vi "FPGA cRIOMain_v5.vi"() -> ()   [LabVIEW 2019]
doc: "Main FPGA VI\nUse the bitfile generated by this VI in the real-time code.\n\nv5: Use 16-pt MA filter in AI loop"
uses:
  TypeDefs/AO mode TabCtrl.ctl
  TypeDefs/SamplingModeEnum.ctl
  TypeDefs/AI_channelEnum.ctl
  <vilib>/rvi/Emulation/niFpgaGetClockAttributes.vi
  <vilib>/rvi/Emulation/niFpgaSctlEmulationGetInTimedLoop.vi
  <vilib>/rvi/Emulation/niFpgaEmulationReportErrorSimple.vi
  <vilib>/rvi/eio/common/nirviEmuTemplateMethod_errors.vi
  <vilib>/rvi/Emulation/niFpgaEmulationIsFPGAContextNoSignature.vi
  <vilib>/rvi/DataTransferAndStorage/Container/Common/niFpgaContainerGetUniqueNameForEmu.vi
  <vilib>/rvi/Memory/Memory_Emulation/niFpgaMemoryEmulationCacheClearOnFirstRun.vi
  <vilib>/rvi/Memory/Memory_Emulation/nirvimemoryEmulationManagerCache_MakeExclusive.vi
  <vilib>/rvi/Memory/Memory_Emulation/niFpgaMemoryEmulationValidateCache.vi
  <vilib>/rvi/Memory/Memory_Emulation/nirvimemoryEmulationManagerCache_InsertValue.vi
  <vilib>/Utility/error.llb/Clear Errors.vi
  <vilib>/rvi/Memory/Memory_Emulation/nirvimemoryEmulationManagerCache_ReleaseExclusive.vi
  <vilib>/rvi/Memory/Memory_Emulation/nirvimemoryEmulationManagerCache_GetValue.vi
  <vilib>/rvi/Memory/Memory_Emulation/nirvimemoryEmulationManagerCache_SetValue.vi
  <vilib>/rvi/Emulation/niFpgaProcessEmulError.vi
  <vilib>/rvi/Emulation/niFpgaCriticalErrorInLSC.vi
  <vilib>/rvi/errors/niFpgaSetErrorForExecOnDevCompSimple.vi
  <vilib>/rvi/eio/common/nirviEmuReportErrorAndStop.vi
  <vilib>/rvi/FIFO/Fifo_Resource/nirvififoEmulationSetSize.vi
  <vilib>/rvi/FIFO/Fifo_Resource/nirviFifoEmulationQueueMgr.vi
  <instcachedir>/0/nirviFifoEmulationQueueMgr_E5CAEC123FF24DC58D834DCA3CDAA9B5.lvgen/nirviFifoEmulationQueueMgr_E5CAEC123FF24DC58D834DCA3CDAA9B5_006.vi
  <vilib>/rvi/FIFO/Fifo_Resource/nirvififoEmulationCreateLock.vi
  <vilib>/rvi/FIFO/Fifo_Resource/nirvififoEmulationObtainLock.vi
  <vilib>/rvi/FIFO/Fifo_Resource/nirvififoEmulationReleaseLock.vi
  <vilib>/rvi/occurrence/nirviWaitOnOccurrenceBase.vi
  <vilib>/rvi/errors/nirviReportUnexpectedCaseInternalError.vi
  <vilib>/rvi/errors/nirviReportUnexpectedCaseInternalError (U32).vi
  <vilib>/rvi/FIFO/Fifo_Resource/nirvififoEmulationDetermineInputValidOut.vi
  <vilib>/eio/EIONode/EIONode.xnode
  <vilib>/rvi/DataTransferAndStorage/Container/XNode/niFpgaContainer.xnode
  <vilib>/rvi/DataTransferAndStorage/Register/Emulation/niFpgaRegisterEmulation.vi
  <vilib>/rvi/FIFO/Fifo_Resource/nirvififoEmulationRead.vi
  <vilib>/rvi/Analysis/measure/butterworth/XNode/niFpgaButterworthFilter.xnode
  <vilib>/rvi/FXPMathLib/FxpMul/XNode/nifxpmath_Multiplier.xnode
  <vilib>/rvi/FIFO/Fifo_Resource/nirvififoEmulationWrite.vi
  FPGA functions/FPGA functions.lvlib
  <vilib>/rvi/FXPMathLib/sim/FxpSim.dll
panel:
  out "AI Processing\nLoop Rate to high?":bool
  in  "AI Process Time [ticks]":u32=121
  in  "Select Channel":T1
  out "Unable to\nsample at desired\nSample Rate?":bool
  out "Processing Loop time [ticks]":u32
  in  "Scaled Butterworth Coeffs":i32[](array[numeric])=[-1036986264, 2110353124, 93741, -1058362983, 2131726043, 94691]
  in  "Sampling Mode":T2
  in  "AO mode":T3
  in  "AO Out [V]":fxp<+/-,18,5> format="%#.6g"
  in  "AO enable?":bool
  out "AI In [V]":fxp<+/-,26,5> format="%#.6g"
  out "FPGA AO DMA\nOverflow?":bool
  out "Int. Output":fxp<+/-,20,5> format="%.17g"
  out "Raw AI Input":fxp<+/-,24,5> format="%.21g"
  in  "Sample Time [ticks]":u32=121
  out "AO Loop time [ticks]":u32
  out "AI Loop time [ticks]":u32
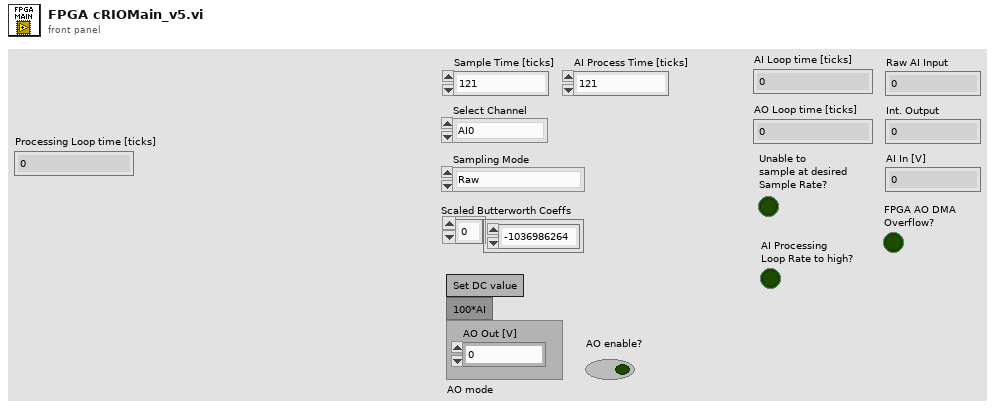
[diagram p1: front panel]
types:
  T1 = typedef "AI_channelEnum.ctl" = enum16{"AI0", "AI1", "AI2", "AI3"}
  T2 = typedef "SamplingModeEnum.ctl" = enum16{"Raw", "M64 (ReSpl)", "M128 (ReSpl)", "4pt MA (AI) + M64 (ReSpl)", "LPF (Proc.)", "4pt MA (AI) + LPF (Proc.)", "4pt MA (Proc.) + LPF (Proc.)"}
  T3 = typedef "AO mode TabCtrl.ctl" = enum32{"Set DC value", "100*AI"}
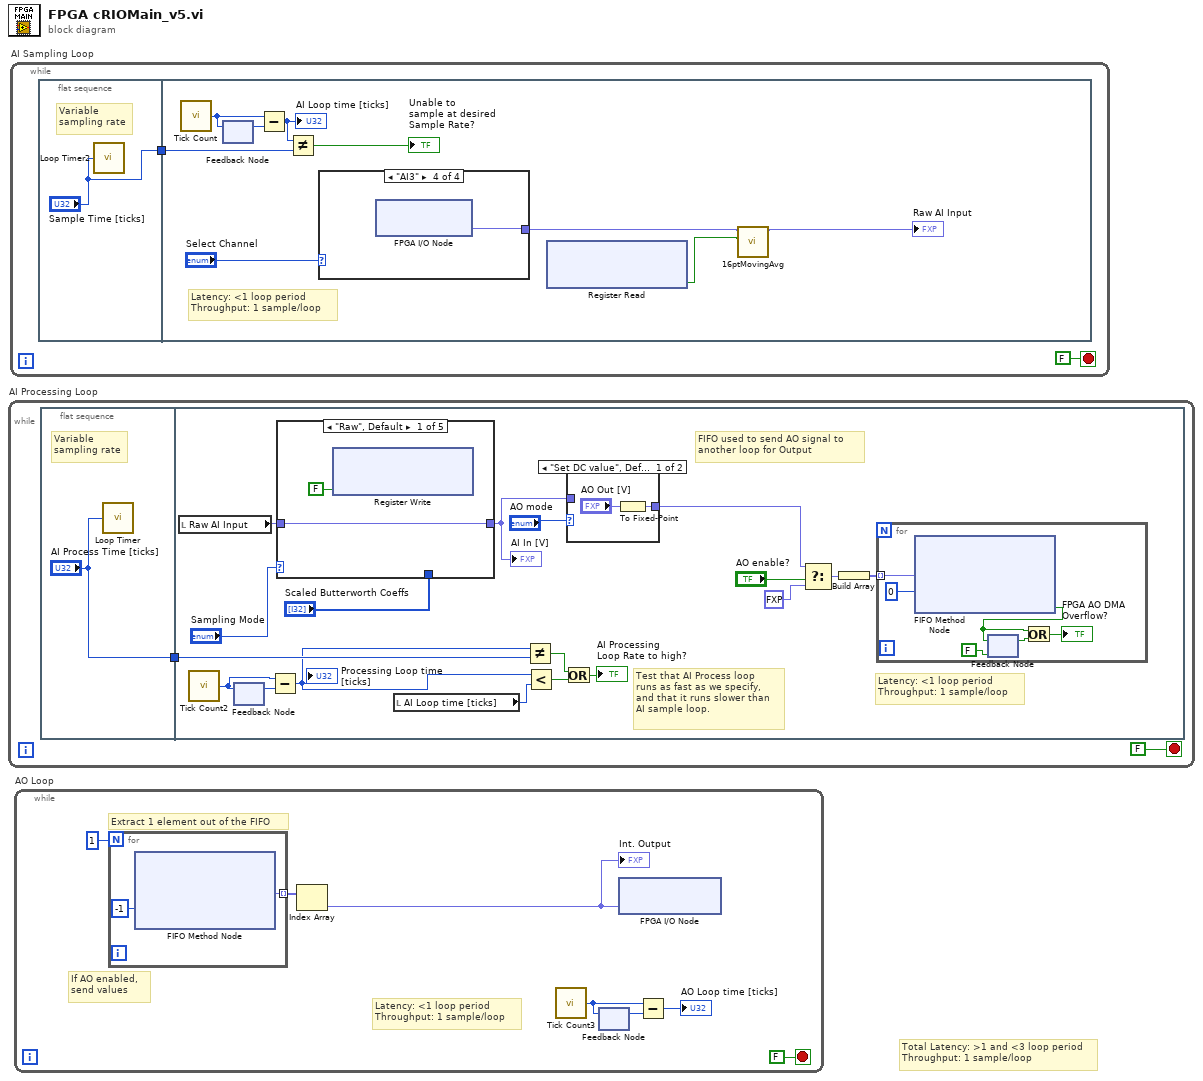
[diagram p0: block diagram]
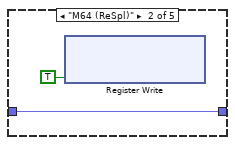
[diagram p2: hidden frame]
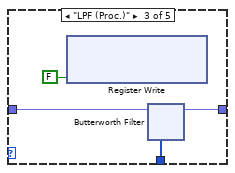
[diagram p3: hidden frame]
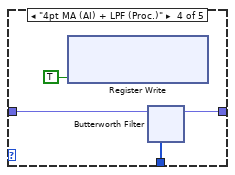
[diagram p4: hidden frame]
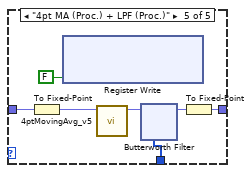
[diagram p5: hidden frame]
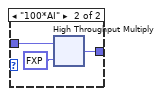
[diagram p6: hidden frame]
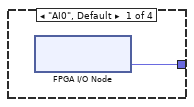
[diagram p7: hidden frame]
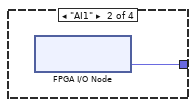
[diagram p8: hidden frame]
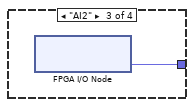
[diagram p9: hidden frame]
diagram:
  # "Total Latency: >1 and <3 loop period\nThroughput: 1 sample/loop"
  n1 = while "AI Processing Loop" {
    stop <- FALSE stop-if-true
    n2 = flat-sequence {
      tunnel: ["AI Process Time [ticks]"] -> w1
      tunnel: w1 -> [w5]
      frame #0 {
        # "Variable\nsampling rate"
        n3 = call "Loop Timer"("Count(Ticks)"="AI Process Time [ticks]") -> ()  [unwired: 1 out]
      }
      frame #1 {
        # "Test that AI Process loop\nruns as fast as we specify,\nand that it runs slower than \nAI sample loop."
        # "Latency: <1 loop period\nThroughput: 1 sample/loop"
        # "FIFO used to send AO signal to \nanother loop for Output"
        n4 = local read "Raw AI Input"() -> (w9:fxp<+/-,24,5>)
        n5 = call "Tick Count2"() -> ("Tick Count(Ticks)"=w20:u32)
        n6 = feedback #1() -> (w21:u32)  [unwired: 1 in]
        n7 = feedback-in #1(w20) -> ()
        n8 = Subtract(x=w20, y=w21) -> (x-y=w4:u32)
        "Processing Loop time [ticks]" <- w4
        n9 = case shown="\"Raw\", Default" "Sampling Mode" {
          tunnel: "Scaled Butterworth Coeffs" -> [_ _ w29 w41 w56]
          tunnel: [w22 w24 w28 w40 w50] -> w18
          tunnel: w9 -> [w22 w24 w26 w38 w53]
          frame "Raw", Default {
            n10 = xnode ("Register Write")("Data"=FALSE) -> ()  [unwired: 1 in, 1 out]
          }
          frame "M64 (ReSpl)" {
            n11 = xnode ("Register Write")("Data"=TRUE) -> ()  [unwired: 1 in, 1 out]
          }
          frame "LPF (Proc.)" {
            n12 = xnode ("Register Write")("Data"=FALSE) -> ()  [unwired: 1 in, 1 out]
            n13 = xnode "Butterworth Filter"("input data"=w26, "scaled coefficients"=w29) -> ("output data"=w28:fxp<+/-,24,5>)  [unwired: 1 in]
          }
          frame "4pt MA (AI) + LPF (Proc.)" {
            n14 = xnode ("Register Write")("Data"=TRUE) -> ()  [unwired: 1 in, 1 out]
            n15 = xnode "Butterworth Filter"("input data"=w38, "scaled coefficients"=w41) -> ("output data"=w40:fxp<+/-,24,5>)  [unwired: 1 in]
          }
          frame "4pt MA (Proc.) + LPF (Proc.)" {
            n16 = To Fixed-Point(number=w53) -> (fixed-point=w54:fxp<+/-,24,5>)  [unwired: 1 in]
            n17 = xnode ("Register Write")("Data"=FALSE) -> ()  [unwired: 1 in, 1 out]
            n18 = call "4ptMovingAvg_v5.vi"("Raw input"=w54) -> ("Avg. output"=w55:fxp<+/-,25,5>)  [unwired: 10 in]
            n19 = xnode "Butterworth Filter"("input data"=w55, "scaled coefficients"=w56) -> ("output data"=w51:fxp<+/-,25,5>)  [unwired: 1 in]
            n20 = To Fixed-Point(number=w51) -> (fixed-point=w50:fxp<+/-,26,5>)  [unwired: 1 in]
          }
        }
        "AI In [V]" <- w18
        n21 = local read "AI Loop time [ticks]"() -> (w10:u32)
        n22 = Not Equal?(x=w4, y=w5) -> (x != y?=w7:bool)
        n23 = Less?(x=w4, y=w10) -> (x < y?=w6:bool)
        n24 = Or(x=w7, y=w6) -> (x .or. y?=→"AI Processing\nLoop Rate to high?":bool)
        n25 = case shown="\"Set DC value\", Default" "AO mode" {
          tunnel: [w66 w67] -> w14
          tunnel: w18 -> [_ w69]
          frame "Set DC value", Default {
            n26 = To Fixed-Point(number="AO Out [V]") -> (fixed-point=w66:fxp<+/-,20,5>)  [unwired: 1 in]
          }
          frame "100*AI" {
            n27 = xnode ("High Throughput Multiply")("x"=w69, "y"=fxp<+,5,7> 100.0) -> ("x*y"=w67:fxp<+/-,20,5>)
          }
        }
        n28 = Select(t=w14, s="AO enable?", f=fxp<+/-,20,5> 0.0) -> (s? t:f=w19:fxp<+/-,20,5>)
        n29 = Build Array(w19) -> (w13:fxp<+/-,20,5>[])
        n30 = for {
          tunnel: w13 -> [w70] mode=indexing
          n31 = xnode ("FIFO Method Node")("Element"=w70, "Timeout"=0) -> ("Timed Out?"=w71:bool)  [unwired: 1 in, 1 out]
          n32 = feedback-in #2(w71) -> ()
          n33 = feedback #2(FALSE ("Timed Out?")) -> (w74:bool)
          n34 = Or(x=w71, y=w74) -> (x .or. y?=→"FPGA AO DMA\nOverflow?":bool)
        }
      }
    }
  }
  n35 = while "AI Sampling Loop" {
    stop <- FALSE stop-if-true
    n36 = flat-sequence {
      tunnel: ["Sample Time [ticks]"] -> w76
      tunnel: w76 -> [w84]
      frame #0 {
        # "Variable\nsampling rate"
        n37 = call "Loop Timer2"("Count(Ticks)"="Sample Time [ticks]") -> ()  [unwired: 1 out]
      }
      frame #1 {
        # "Latency: <1 loop period\nThroughput: 1 sample/loop"
        n38 = call "Tick Count"() -> ("Tick Count(Ticks)"=w87:u32)
        n39 = feedback #3() -> (w86:u32)  [unwired: 1 in]
        n40 = feedback-in #3(w87) -> ()
        n41 = Subtract(x=w87, y=w86) -> (x-y=w85:u32)
        "AI Loop time [ticks]" <- w85
        n42 = Not Equal?(x=w85, y=w84) -> (x != y?=→"Unable to\nsample at desired\nSample Rate?":bool)
        n43 = case shown="\"AI3\"" "Select Channel" {
          tunnel: [w88 w89 w90 w91] -> w80
          frame "AI0", Default {
            n44 = xnode "FPGA I/O Node"() -> ("Mod4/AI0"=w88:fxp<+/-,24,5>)  [unwired: 1 in, 1 out]
          }
          frame "AI1" {
            n45 = xnode "FPGA I/O Node"() -> ("Mod4/AI1"=w89:fxp<+/-,24,5>)  [unwired: 1 in, 1 out]
          }
          frame "AI2" {
            n46 = xnode "FPGA I/O Node"() -> ("Mod4/AI2"=w90:fxp<+/-,24,5>)  [unwired: 1 in, 1 out]
          }
          frame "AI3" {
            n47 = xnode "FPGA I/O Node"() -> ("Mod4/AI3"=w91:fxp<+/-,24,5>)  [unwired: 1 in, 1 out]
          }
        }
        n48 = xnode ("Register Read")() -> ("Data"=w79:bool)  [unwired: 1 in, 1 out]
        n49 = call "16ptMovingAvg.vi"("Enable?"=w79, "Raw input"=w80) -> ("Output"=→"Raw AI Input":fxp<+/-,24,5>)  [unwired: 9 in]
      }
    }
  }
  n50 = while "AO Loop" {
    stop <- FALSE stop-if-true
    # "Latency: <1 loop period\nThroughput: 1 sample/loop"
    # "If AO enabled, \nsend values"
    # "Extract 1 element out of the FIFO"
    n51 = for {
      N: 1 -> [_]
      tunnel: [w100] -> w94 mode=indexing
      n52 = xnode ("FIFO Method Node")("Timeout"=-1) -> ("Element"=w100:fxp<+/-,20,5>)  [unwired: 1 in, 2 out]
    }
    n53 = Index Array(array=w94) -> (element=w92:fxp<+/-,20,5>)  [unwired: 1 in]
    "Int. Output" <- w92
    n54 = call "Tick Count3"() -> ("Tick Count(Ticks)"=w97:u32)
    n55 = feedback #4() -> (w96:u32)  [unwired: 1 in]
    n56 = feedback-in #4(w97) -> ()
    n57 = xnode "FPGA I/O Node"("Mod3/AO1"=w92) -> ()  [unwired: 1 in, 1 out]
    n58 = Subtract(x=w97, y=w96) -> (x-y=→"AO Loop time [ticks]":u32)
  }
